vi "Time to String.vi"(1 "Time Stamp":timestamp) -> (0 "date/time string":string)   [LabVIEW 2015, in "Exposure Process.lvlib"]
uses:
  Exposure Process.lvlib
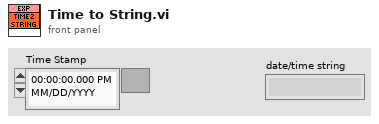
[diagram p1: front panel]
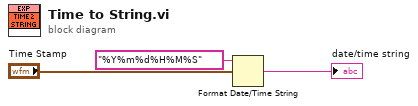
[diagram p0: block diagram]
diagram:
  n1 = Format Date/Time String(time format string (%c)="%Y%m%d%H%M%S", seconds (now)="Time Stamp") -> (date/time string=→"date/time string":string)  [unwired: 1 in]
